vi "Set Output.vi"(8 "error in (no error)":errorcluster, 9 "Enable?":bool, 10 "Output Channel":T1, 11 "LINX-AutomationHat in":refnum<class "LINX-AutomationHat.lvclass">) -> (0 "error out":errorcluster, 3 "LINX-AutomationHat out":refnum<class "LINX-AutomationHat.lvclass">)   [LabVIEW 2020, in "LINX-AutomationHat.lvclass"]
doc: "Controls the relay and sinking outputs."
uses:
  LINX-AutomationHat.lvclass
  Output Channels.ctl
  LEDs.ctl
  GPIO/LINX GPIO.lvclass
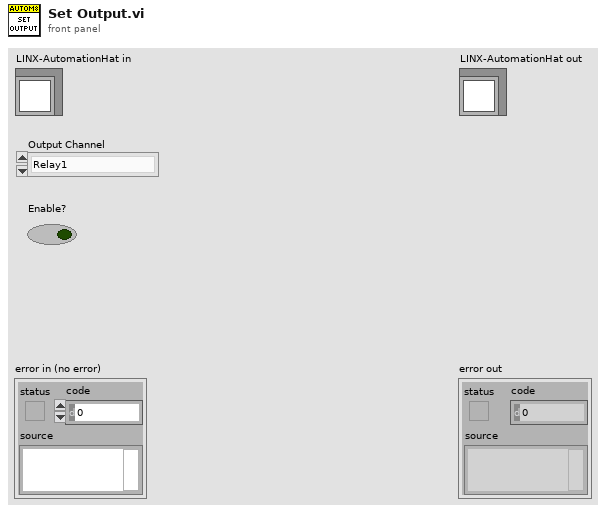
[diagram p1: front panel]
types:
  T1 = typedef "LINX-AutomationHat.lvclass/Output Channels.ctl" = enum16{"Relay1", "Relay2", "Relay3", "Output1", "Output2", "Output3"}
  T2 = typedef "LINX-AutomationHat.lvclass/LEDs.ctl" = enum16{"All", "ADC1", "ADC2", "ADC3", "Output1", "Output2", "Output3", "Relay1NO", "Relay1NC", "Relay2NO", "Relay2NC", "Relay3NO", "Relay3NC", "Input3", "Input2", "Input1", "Warn", "Comms", "Power"}
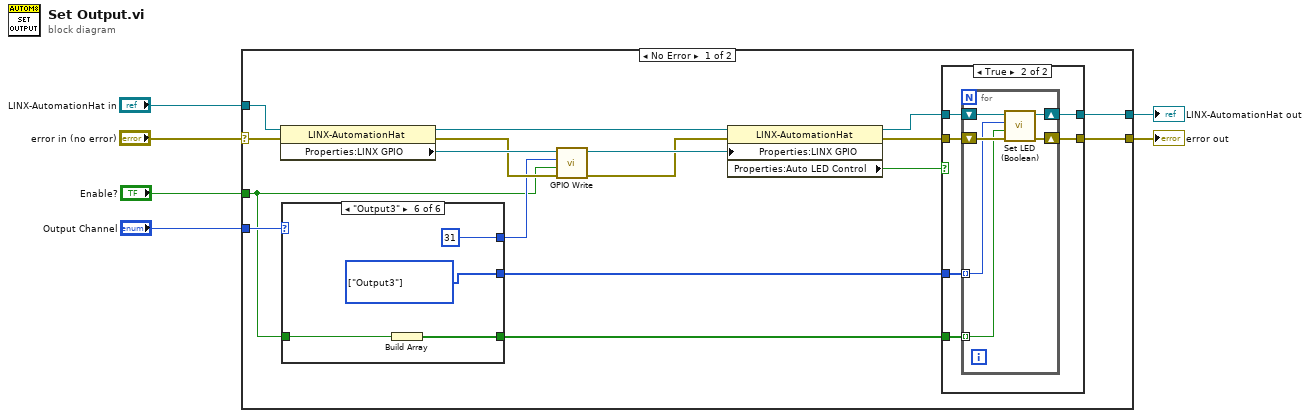
[diagram p0: block diagram]
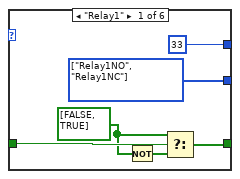
[diagram p3: hidden frame]
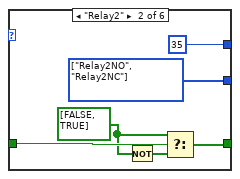
[diagram p4: hidden frame]
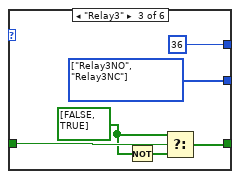
[diagram p5: hidden frame]
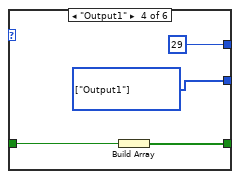
[diagram p6: hidden frame]
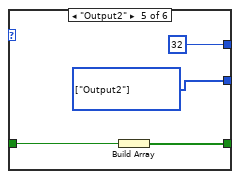
[diagram p7: hidden frame]
diagram:
  n1 = case shown="No Error" "error in (no error)" {
    selector: "error in (no error)" -> [w13 w69]
    tunnel: [w20 w69] -> w5
    tunnel: [w23 w68] -> w3
    tunnel: "LINX-AutomationHat in" -> [w19 w68]
    tunnel: "Enable?" -> [w7 _]
    tunnel: "Output Channel" -> [w12 _]
    frame No Error {
      n2 = property class="LINX-AutomationHat"(reference=w19, error in=w13) -> (reference out=w18:refnum<class "LINX-AutomationHat.lvclass">, error out=w15:errorcluster, "Properties:LINX GPIO"=w17:refnum<class "LINX GPIO.lvclass">)
      n3 = case shown="\"Output3\"" w12 {
        tunnel: [u8 33 ("DO Channel") u8 35 ("DO Channel") u8 36 ("DO Channel") u8 29 ("DO Channel") u8 32 ("DO Channel") u8 31 ("DO Channel")] -> w11
        tunnel: [w42 w48 w54 w58 w62 w66] -> w10
        tunnel: [w38 w44 w50 w57 w61 w65] -> w9
        tunnel: w7 -> [w41 w47 w53 w56 w60 w64]
        frame "Relay1" {
          w40 = bool[] [FALSE, TRUE]
          w42 = T2[] [enum."Relay1NO", enum."Relay1NC"] items=["All", "ADC1", "ADC2", "ADC3", "Output1", "Output2", "Output3", "Relay1NO", "Relay1NC", "Relay2NO", "Relay2NC", "Relay3NO", "Relay3NC", "Input3", "Input2", "Input1", "Warn", "Comms", "Power"] ("LED Selector")
          n4 = Not(x=w40) -> (.not. x?=w39:bool[])
          n5 = Select(t=w40, s=w41, f=w39) -> (s? t:f=w38:bool[])
        }
        frame "Relay2" {
          w46 = bool[] [FALSE, TRUE]
          w48 = T2[] [enum."Relay2NO", enum."Relay2NC"] items=["All", "ADC1", "ADC2", "ADC3", "Output1", "Output2", "Output3", "Relay1NO", "Relay1NC", "Relay2NO", "Relay2NC", "Relay3NO", "Relay3NC", "Input3", "Input2", "Input1", "Warn", "Comms", "Power"] ("LED Selector")
          n6 = Not(x=w46) -> (.not. x?=w45:bool[])
          n7 = Select(t=w46, s=w47, f=w45) -> (s? t:f=w44:bool[])
        }
        frame "Relay3" {
          w52 = bool[] [FALSE, TRUE]
          w54 = T2[] [enum."Relay3NO", enum."Relay3NC"] items=["All", "ADC1", "ADC2", "ADC3", "Output1", "Output2", "Output3", "Relay1NO", "Relay1NC", "Relay2NO", "Relay2NC", "Relay3NO", "Relay3NC", "Input3", "Input2", "Input1", "Warn", "Comms", "Power"] ("LED Selector")
          n8 = Not(x=w52) -> (.not. x?=w51:bool[])
          n9 = Select(t=w52, s=w53, f=w51) -> (s? t:f=w50:bool[])
        }
        frame "Output1" {
          w58 = T2[] [enum."Output1"] items=["All", "ADC1", "ADC2", "ADC3", "Output1", "Output2", "Output3", "Relay1NO", "Relay1NC", "Relay2NO", "Relay2NC", "Relay3NO", "Relay3NC", "Input3", "Input2", "Input1", "Warn", "Comms", "Power"] ("LED Selector")
          n10 = Build Array(w56) -> (w57:bool[])
        }
        frame "Output2" {
          w62 = T2[] [enum."Output2"] items=["All", "ADC1", "ADC2", "ADC3", "Output1", "Output2", "Output3", "Relay1NO", "Relay1NC", "Relay2NO", "Relay2NC", "Relay3NO", "Relay3NC", "Input3", "Input2", "Input1", "Warn", "Comms", "Power"] ("LED Selector")
          n11 = Build Array(w60) -> (w61:bool[])
        }
        frame "Output3" {
          w66 = T2[] [enum."Output3"] items=["All", "ADC1", "ADC2", "ADC3", "Output1", "Output2", "Output3", "Relay1NO", "Relay1NC", "Relay2NO", "Relay2NC", "Relay3NO", "Relay3NC", "Input3", "Input2", "Input1", "Warn", "Comms", "Power"] ("LED Selector")
          n12 = Build Array(w64) -> (w65:bool[])
        }
      }
      n13 = call-dynamic "GPIO Write.vi"("error in (no error)"=w15, "Output Value"=w7, "DO Channel"=w11, "LINX GPIO in"=w17) -> ("error out"=w14:errorcluster, "LINX GPIO out"=w16:refnum<class "LINX GPIO.lvclass">)  [unwired: 6 in]
      n14 = property class="LINX-AutomationHat"(reference=w18, error in=w14, "Properties:LINX GPIO"=w16) -> (reference out=w22:refnum<class "LINX-AutomationHat.lvclass">, error out=w21:errorcluster, "Properties:Auto LED Control"=w8:bool)
      n15 = case shown="True" w8 {
        tunnel: [w25 w31] -> w23
        tunnel: w22 -> [w25 w30]
        tunnel: w21 -> [w24 w29]
        tunnel: [w24 w28] -> w20
        tunnel: w10 -> [_ w27]
        tunnel: w9 -> [_ w26]
        frame False {
        }
        frame True {
          n16 = for {
            shift-right: [w37] -> w31
            shift-left: w30 -> [w36]
            shift-right: [w34] -> w28
            shift-left: w29 -> [w35]
            tunnel: w27 -> [w33] mode=indexing
            tunnel: w26 -> [w32] mode=indexing
            n17 = call-dynamic "Set LED (Boolean).vi"("error in (no error)"=w35, "Enable"=w32, "LED Selector"=w33, "LINX-AutomationHat in"=w36) -> ("error out"=w34:errorcluster, "LINX-AutomationHat out"=w37:refnum<class "LINX-AutomationHat.lvclass">)  [unwired: 6 in]
          }
        }
      }
    }
    frame Error {
    }
  }
  "error out" <- w5
  "LINX-AutomationHat out" <- w3
